vi "ScanForMinimum.vi"(0 "TLCamera reference in":refnum<k24>, 1 "MotorController in":refnum<class "MotorController.lvclass">, 2 "Exposure (us)":u32, 5 "Axis":T1, 7 "Start Angle (deg)":i32, 9 "Stop Angle (deg)":i32, 11 "Error In":errorcluster) -> (3 "MotorController Out":refnum<class "MotorController.lvclass">, 4 "TLCamera reference out":refnum<k24>, 6 "Angles":i32[](array[numeric]), 8 "Amplitudes":dbl[](array[numeric]), 10 "Angle of Minimum":i32, 15 "Error Out":errorcluster)   [LabVIEW 2019]
uses:
  Axes_enum_typedef.ctl
  MotorController.lvclass
  C:/Users/jleeman/git_repos/CAxis_Machine/C-Axis LabView Controller/Library_X64/Thorlabs.TSI.TLCameraInterfaces.dll
  Library_X64/Thorlabs.TSI.TLCameraInterfaces.dll
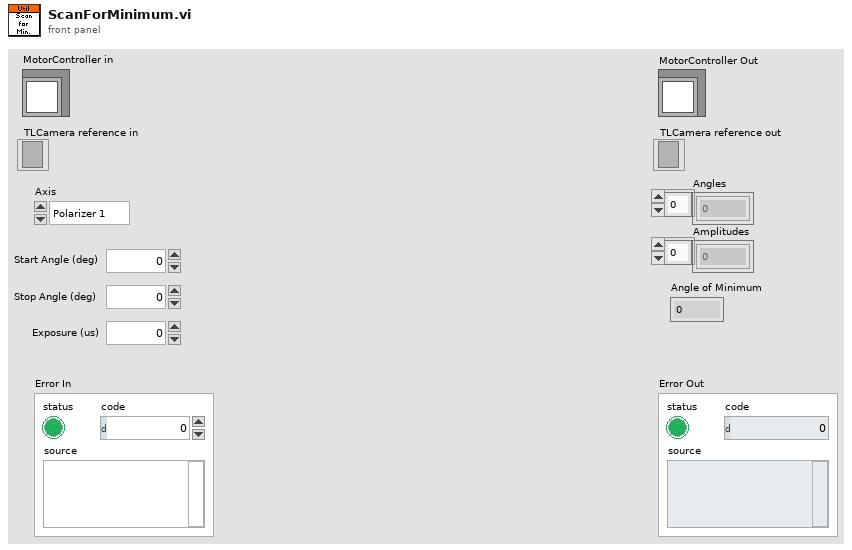
[diagram p1: front panel]
types:
  T1 = typedef "Axes_enum_typedef.ctl" = enum16{"Polarizer 1", "Polarizer 2", "Sample", "Stage"}
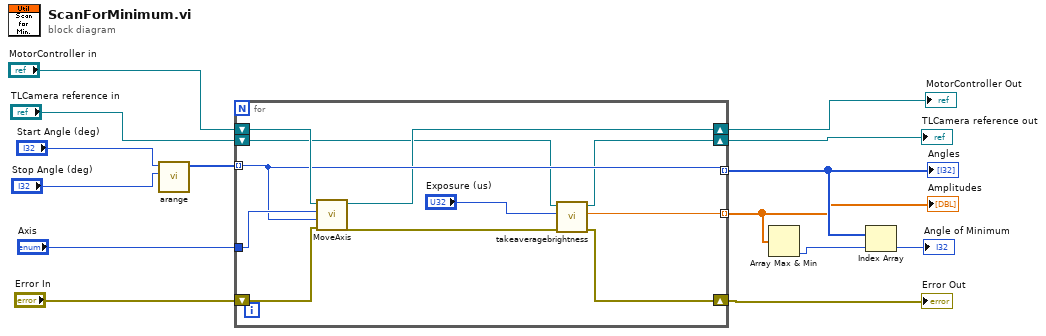
[diagram p0: block diagram]
diagram:
  n1 = call "arange.vi"("Stop"="Stop Angle (deg)", "Start"="Start Angle (deg)") -> ("Array"=w12:i32[])  [unwired: 9 in]
  n2 = for {
    tunnel: w12 -> [w23] mode=indexing
    tunnel: "Axis" -> [w25]
    tunnel: [w23] -> w9 mode=indexing
    shift-right: [w21] -> w7
    shift-left: "MotorController in" -> [w24]
    shift-right: [w19] -> w5
    shift-left: "TLCamera reference in" -> [w20]
    shift-right: [w18] -> w2
    shift-left: "Error In" -> [w22]
    tunnel: [w15] -> w1 mode=indexing
    n3 = call "MoveAxis.vi"("error in (no error)"=w22, "Position"=w23, "Axis"=w25, "MotorController in"=w24) -> ("error out"=w17:errorcluster, "MotorController out"=w21:refnum<class "MotorController.lvclass">)  [unwired: 6 in]
    n4 = call "takeaveragebrightness.vi"("Error In"=w17, "Exposure (us)"="Exposure (us)", "TLCamera reference in"=w20) -> ("Error Out"=w18:errorcluster, "brightness"=w15:dbl, "TLCamera reference out"=w19:refnum<k24>)  [unwired: 6 in]
  }
  "Angles" <- w9
  "MotorController Out" <- w7
  "TLCamera reference out" <- w5
  "Amplitudes" <- w1
  "Error Out" <- w2
  n5 = Array Max & Min(array=w1) -> (min index (indices)=w4:i32)  [unwired: 3 out]
  n6 = Index Array(array=w9, index=w4) -> (element=→"Angle of Minimum":i32)
